vi "Period Curve and Skew Edge Triangular Generator.vi"() -> ()   [LabVIEW 2014]
uses:
  <vilib>/Analysis/Matrix/Datatypes/RealMatrix.ctl
  <vilib>/Analysis/Matrix/NI_Matrix.lvlib
panel:
  in  "S-G Polynomial Order":i32=3
  in  "S-G Side Points":i32=15
  in  "Signals Matrix":T1
  in  "Triangular edge":enum16{"Rising", "Falling"}(ring)
  in  "Interpolation Method":i32(ring)=2 items=["nearest", "linear", "spline", "cubic Hermite", "Lagrange"]
  out "Skew Triangular Edge":dbl[](graph)
  out "Period curve":dbl[](graph)
  # "Smoothing: Savitzky-Golay Parameters"
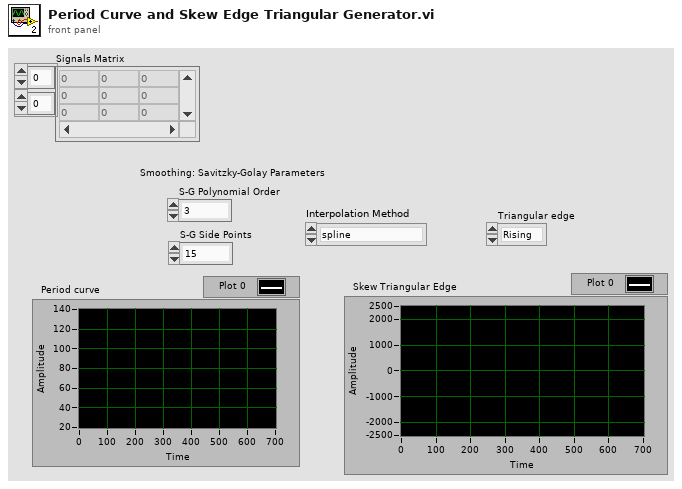
[diagram p1: front panel]
types:
  T1 = typedef "NI_Matrix.lvlib/RealMatrix.ctl" = dbl[][]
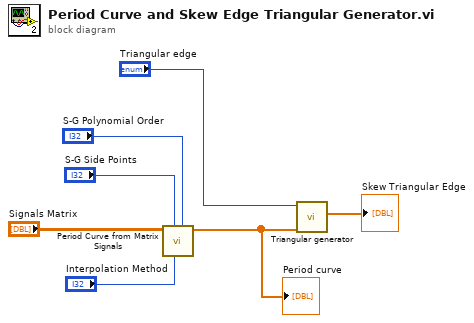
[diagram p0: block diagram]
diagram:
  n1 = call "Period Curve from Matrix Signals.vi"("S-G Polynomial Order"="S-G Polynomial Order", "Interpolation Method"="Interpolation Method", "S-G Side Points"="S-G Side Points", "Signals Matrix"="Signals Matrix") -> ("Period Length Curve"=w6:dbl[])  [unwired: 6 in, 1 out]
  "Period curve" <- w6
  n2 = call "Triangular generator.vi"("Sample values"=w6, "Triangular edge"="Triangular edge") -> ("Skew Triangular"=→"Skew Triangular Edge":dbl[])  [unwired: 9 in]
